vi "tell controller status.vi"(0 "VISA Handle in":refnum<visa-resource-name>, 5 "Axis in":i32=1, 11 "error in":errorcluster) -> (2 "TimeoutFlag":bool, 4 "VISA Handle out":refnum<visa-resource-name>, 6 "Axis out":i32=1, 8 "Controller's error":string, 10 "Controller's state":string, 15 "error out":errorcluster)   [LabVIEW 2018]
doc: "This VI return the controller's state and the controller's error.\nThe controller's error is composed to 4 digits (abcd) coded in hexadecimal, each bit of the error byte is described bellow :\n- Digit d bit 0 : negative end of run\n- Digit d bit 1 : positive end of run \n- Digit d bit 2 : peak current limit\n- Digit d bit 3 : rms current limit\n- Digit c bit 0 : short circuit detection\n- Digit c bit 1 : following error\n- Digit c bit 2 : time out homing\n- Digit c bit 3 : bad SmartStage\n- Digit b bit 0 : D.C voltage too low\n- Digit b bit 1 : 80W output power exceeded\n\nController state values : \n- 0A : NOT REFERENCE from reset\n- 0B : NOT REFERENCE from HOMING mode\n- 0C : NOT REFERENCE from CONFIGURATION mode\n- 0D : NOT REFERENCE from DISABLE mode\n- 0E : NOT REFERENCE from READY mode\n- 0F : NOT REFERENCE from MOVING mode\n- 10 : NOT REFERENCE from Smartstage error\n- 14 : CONFIGURATION\n- 1E : HOMING\n- 28 : MOVING\n- 32 : READY from HOMING mode\n- 33 : READY from MOVING mode\n- 34 : READY from DISABLE mode\n- 3C : DISABLE from READY mode\n- 3D : DISABLE from MOVING mode"
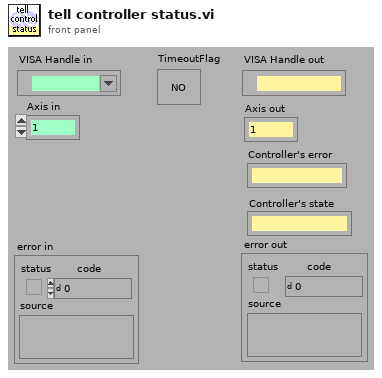
[diagram p1: front panel]
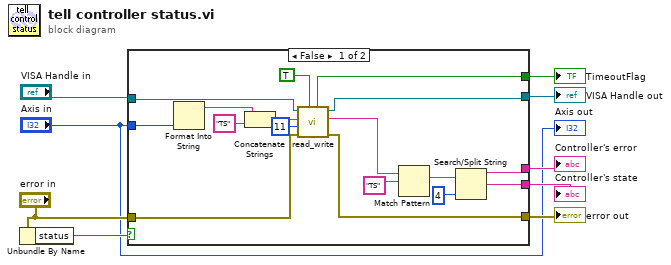
[diagram p0: block diagram]
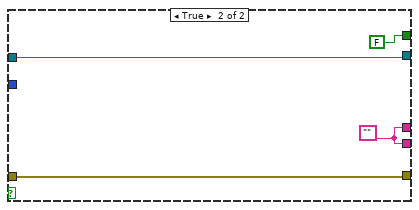
[diagram p2: hidden frame]
diagram:
  n1 = Unbundle By Name("error in") -> ("status"=w7:bool)
  n2 = case shown="False" w7 {
    tunnel: [w22 w30] -> w9
    tunnel: [w21 w29] -> w8
    tunnel: "VISA Handle in" -> [w25 w30]
    tunnel: "error in" -> [w23 w29]
    tunnel: [w20 FALSE ("TimeoutFlag")] -> w5
    tunnel: "Axis in" -> [w11 _]
    tunnel: [w13 w27] -> w4
    tunnel: [w12 w27] -> w3
    frame False {
      n3 = Format Into String(w11) -> (resulting string=w18:string)  [unwired: 3 in, 1 out]
      n4 = Concatenate Strings(w18, "TS" ("string")) -> (w24:string)
      n5 = call "read_write.vi"("Query?"=TRUE, "error in"=w23, "Bytes to read"=11, "Command"=w24, "VISA handle in"=w25) -> ("error out"=w21:errorcluster, "Response"=w17:string, "VISA handle out"=w22:refnum<visa-resource-name>, "TimeoutFlag"=w20:bool)  [unwired: 1 in]
      n6 = Match Pattern(string=w17, regular expression="TS" ("expression")) -> (after substring=w15:string)  [unwired: 1 in, 3 out]
      n7 = Search/Split String(string=w15, offset (0)=4) -> (substring before match=w13:string, match + rest of string=w12:string)  [unwired: 1 in, 1 out]
    }
    frame True {
      w27 = ""
    }
  }
  "VISA Handle out" <- w9
  "error out" <- w8
  "TimeoutFlag" <- w5
  "Controller's state" <- w3
  "Controller's error" <- w4
  "Axis out" <- "Axis in"
